vi "I2C_SCL_DAQ.vi"(2 "SCL_Data":bool) -> ()   [LabVIEW 2022 SP3]
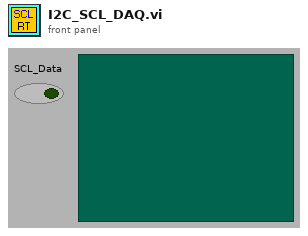
[diagram p1: front panel]
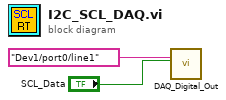
[diagram p0: block diagram]
diagram:
  n1 = call "DAQ_Digital_Out.vi"("Write"="SCL_Data", "Output Chanel"="Dev1/port0/line1") -> ()  [unwired: 9 in, 1 out]
